vi "search_command_from_LUT_and_execute.vi"(2 "parameter_string":string, 3 "input_general_command":string, 4 "input_machine_reference.lvclass":refnum<class "machine.lvclass">) -> (0 "output_specific_command":string, 1 "output_machine_reference.lvclass":refnum<class "machine.lvclass">)   [LabVIEW 2014, in "machine.lvclass"]
uses:
  machine.lvclass
  machine.lvclass/machine.ctl
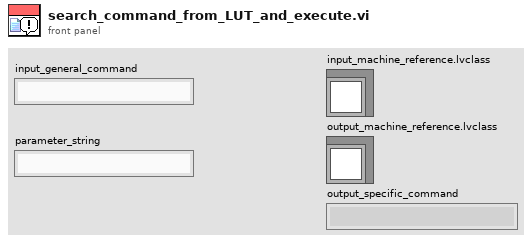
[diagram p1: front panel]
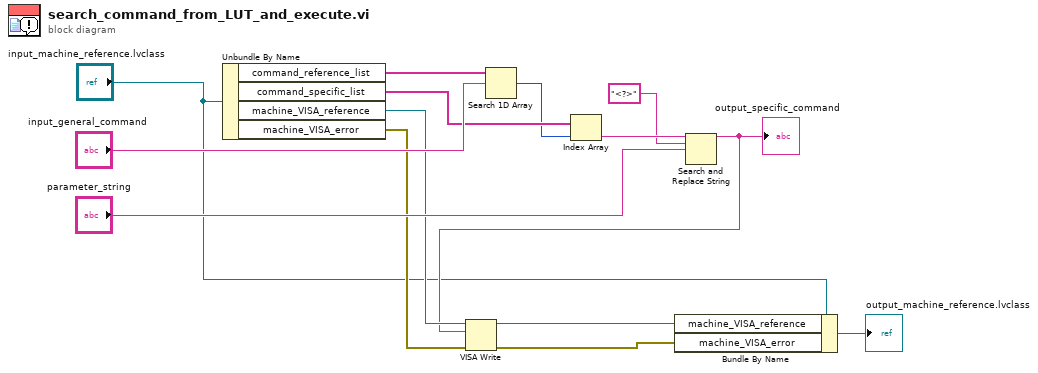
[diagram p0: block diagram]
diagram:
  n1 = Unbundle By Name("input_machine_reference.lvclass") -> ("command_reference_list"=w14:string[], "command_specific_list"=w12:string[], "machine_VISA_reference"=w7:refnum<visa-resource-name>, "machine_VISA_error"=w6:errorcluster)
  n2 = Search 1D Array(1D array=w14, element="input_general_command") -> (index of element=w11:i32)  [unwired: 1 in]
  n3 = Index Array(array=w12, index=w11) -> (element=w10:string)
  n4 = Search and Replace String(input string=w10, search string="<?>", replace string="parameter_string") -> (result string=w5:string)  [unwired: 5 in, 3 out]
  "output_specific_command" <- w5
  n5 = VISA Write(VISA resource name=w7, write buffer=w5, error in (no error)=w6) -> (VISA resource name out=w2:refnum<visa-resource-name>, error out=w1:errorcluster)  [unwired: 1 out]
  n6 = Bundle By Name(cluster="input_machine_reference.lvclass", "machine_VISA_reference"=w2, "machine_VISA_error"=w1) -> (→"output_machine_reference.lvclass":refnum<class "machine.lvclass">)
